vi "InitializeSettings.Do.vi"(8 "error in (no error)":errorcluster, 10 "State Variables":T9, 11 "gRPC Request":T1) -> (0 "error out":errorcluster, 2 "State Variables out":T9, 3 "gRPC Response":T6)   [LabVIEW 2025, in "xnet_can_bus_monitor_api_server_do.lvlib"]
uses:
  xnet_can_bus_monitor_api_server_do.lvlib
  Types/MainProcess.StateVariables.ctl
  Types/XNET.InitialSettings.ctl
  xnet_can_bus_monitor_api_server/RPC Messages/ni_xnet_can_bm_api_ConnectSettings.ctl
  xnet_can_bus_monitor_api_server/RPC Messages/ni_xnet_can_bm_api_CanMode.ctl
  xnet_can_bus_monitor_api_server/RPC Messages/ni_xnet_can_bm_api_Termination.ctl
  xnet_can_bus_monitor_api_server/RPC Messages/ni_xnet_can_bm_api_FdIsoMode.ctl
  xnet_can_bus_monitor_api_server/RPC Messages/ni_xnet_can_bm_api_FilterInfo.ctl
  xnet_can_bus_monitor_api_server/RPC Messages/ni_xnet_can_bm_api_DirectionFilter.ctl
  xnet_can_bus_monitor_api_server/RPC Messages/ni_xnet_can_bm_api_FrameFilter.ctl
  Types/StreamProcess.Refs.ctl
  Types/StreamProcess.VIRef.ctl
  xnet_can_bus_monitor_api_server/RPC Messages/ni_xnet_can_bm_api_InitializeSettingsReply.ctl
  xnet_can_bus_monitor_api_server/RPC Messages/ni_xnet_can_bm_api_Session.ctl
  xnet_can_bus_monitor_api_server/RPC Messages/ni_xnet_can_bm_api_ErrorInfo.ctl
  xnet_can_bus_monitor_api_server/RPC Messages/ni_xnet_can_bm_api_InitializeSettingsRequest.ctl
  <vilib>/xnet/xnet.llb/XNET Create Session (Frame Output Stream).vi
  xnet_can_bus_monitor_api_server/xnet_can_bus_monitor_api_server.lvlib
  <resource>/objmgr/xnet.rc
  <vilib>/numeric/Random Number (Range) U64.vi
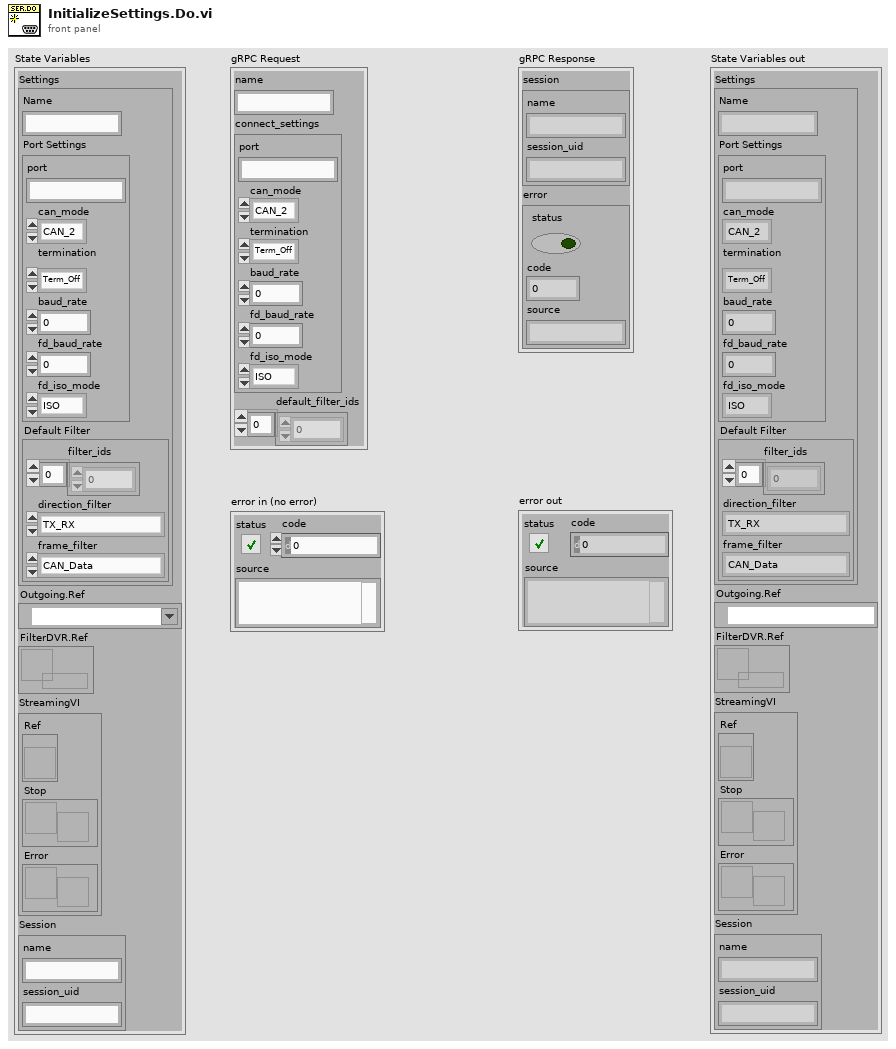
[diagram p1: front panel]
types:
  T1 = typedef "xnet_can_bus_monitor_api_server.lvlib/ni_xnet_can_bm_api_InitializeSettingsRequest.ctl" = cluster{"name":string, "connect_settings":T2, "default_filter_ids":u32[]}
  T2 = typedef "xnet_can_bus_monitor_api_server.lvlib/ni_xnet_can_bm_api_ConnectSettings.ctl" = cluster{"port":string, "can_mode":T3, "termination":T4, "baud_rate":u64, "fd_baud_rate":u64, "fd_iso_mode":T5}
  T3 = typedef "xnet_can_bus_monitor_api_server.lvlib/ni_xnet_can_bm_api_CanMode.ctl" = enum32{"CAN_2", "CAN_FD", "CAN_FD_BRS"}
  T4 = typedef "xnet_can_bus_monitor_api_server.lvlib/ni_xnet_can_bm_api_Termination.ctl" = enum32{"Term_Off", "Term_On"}
  T5 = typedef "xnet_can_bus_monitor_api_server.lvlib/ni_xnet_can_bm_api_FdIsoMode.ctl" = enum32{"ISO", "Non_ISO", "ISO_Legacy"}
  T6 = typedef "xnet_can_bus_monitor_api_server.lvlib/ni_xnet_can_bm_api_InitializeSettingsReply.ctl" = cluster{"session":T7, "error":T8}
  T7 = typedef "xnet_can_bus_monitor_api_server.lvlib/ni_xnet_can_bm_api_Session.ctl" = cluster{"name":string, "session_uid":string}
  T8 = typedef "xnet_can_bus_monitor_api_server.lvlib/ni_xnet_can_bm_api_ErrorInfo.ctl" = errorcluster
  T9 = typedef "xnet_can_bus_monitor_api_server_do.lvlib/MainProcess.StateVariables.ctl" = cluster{"Settings":T10, "Outgoing.Ref":refnum<k21>, "FilterDVR.Ref":refnum<data-value>, "StreamingVI":T14, "Session":T7}
  T10 = typedef "xnet_can_bus_monitor_api_server_do.lvlib/XNET.InitialSettings.ctl" = cluster{"Name":string, "Port Settings":T2, "Default Filter":T11}
  T11 = typedef "xnet_can_bus_monitor_api_server.lvlib/ni_xnet_can_bm_api_FilterInfo.ctl" = cluster{"filter_ids":u32[], "direction_filter":T12, "frame_filter":T13}
  T12 = typedef "xnet_can_bus_monitor_api_server.lvlib/ni_xnet_can_bm_api_DirectionFilter.ctl" = enum32{"TX_RX", "RX", "TX"}
  T13 = typedef "xnet_can_bus_monitor_api_server.lvlib/ni_xnet_can_bm_api_FrameFilter.ctl" = enum32{"CAN_Data", "CAN_Remote", "CAN_Bus_Error", "CAN_2_Data", "CAN_FD_Data", "CAN_FD_BRS_Data", "J1939_Data", "Delay", "Log_Trigger", "Start_Trigger", "All"}
  T14 = typedef "xnet_can_bus_monitor_api_server_do.lvlib/StreamProcess.Refs.ctl" = cluster{"Ref":T15, "Stop":refnum<notifier>, "Error":refnum<notifier>}
  T15 = typedef "xnet_can_bus_monitor_api_server_do.lvlib/StreamProcess.VIRef.ctl" = refnum<vi>
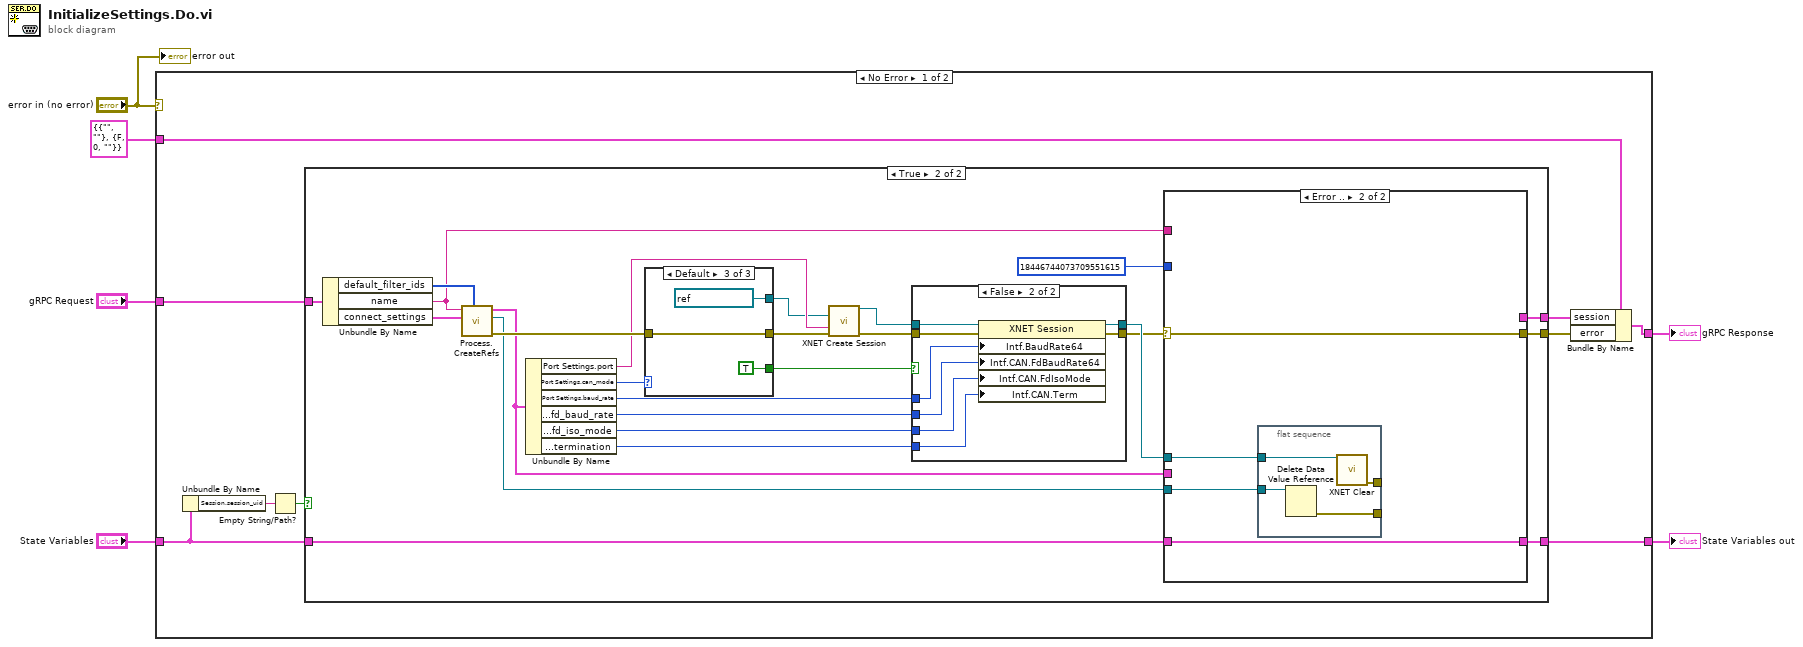
[diagram p0: block diagram]
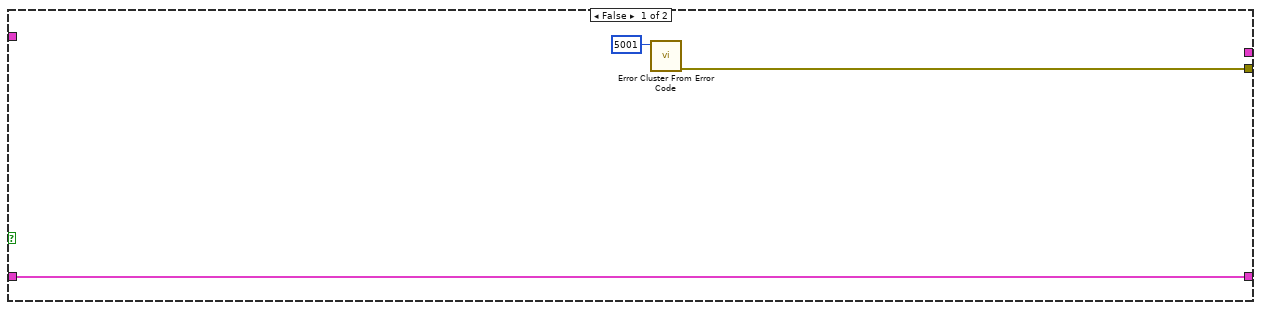
[diagram p2: hidden frame]
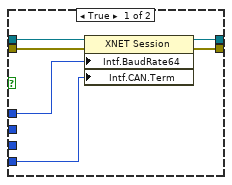
[diagram p3: hidden frame]
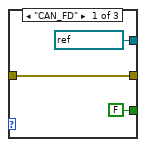
[diagram p4: hidden frame]
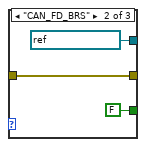
[diagram p5: hidden frame]
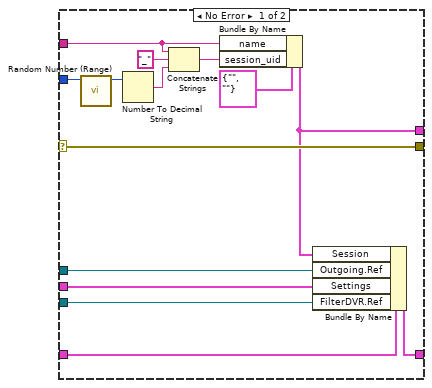
[diagram p6: hidden frame]
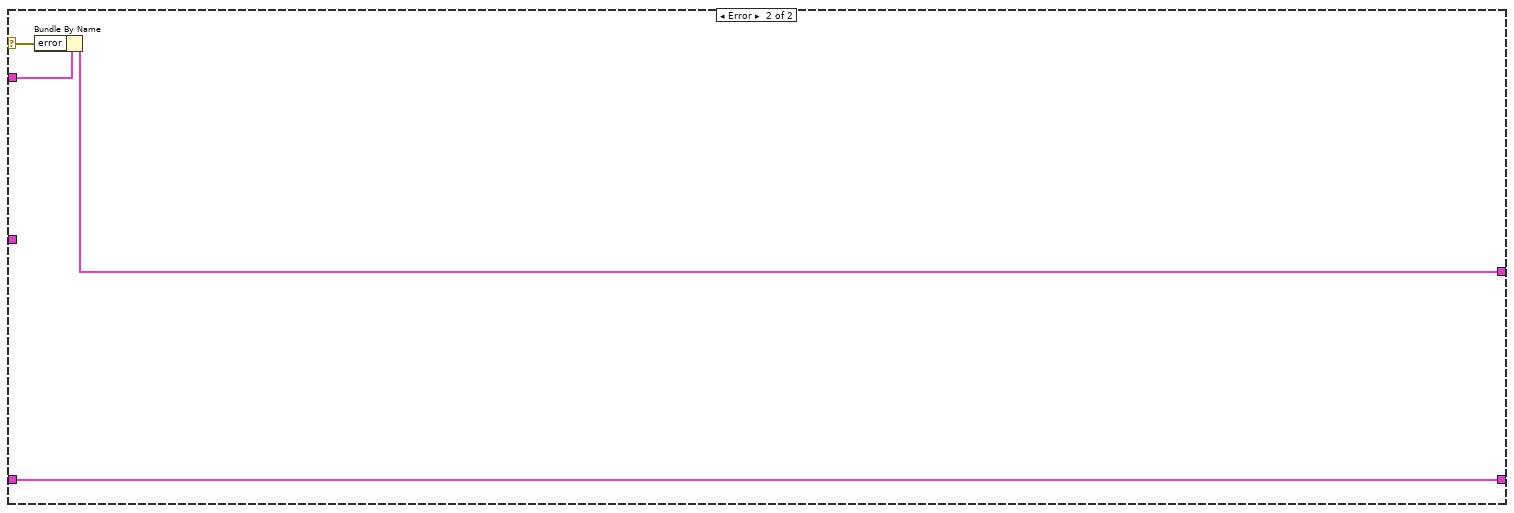
[diagram p7: hidden frame]
diagram:
  n1 = case shown="No Error" "error in (no error)" {
    selector: "error in (no error)" -> [_ w90]
    tunnel: "State Variables" -> [w14 w92]
    tunnel: [w13 w92] -> w5
    tunnel: [w10 w89] -> w4
    tunnel: "gRPC Request" -> [w9 _]
    tunnel: T6 {"session"={"name"="", "session_uid"=""}, "error"={"status"=FALSE, "code"=0, "source"=""}} ("Message Data") -> [w8 w91]
    frame No Error {
      n2 = Unbundle By Name(w14) -> ("Session.session_uid"=w15:string)
      n3 = Empty String/Path?(string/path=w15) -> (empty?=w12:bool)
      n4 = case shown="True" w12 {
        tunnel: w9 -> [_ w43]
        tunnel: [w18 w25] -> w13
        tunnel: [w17 w22] -> w11
        tunnel: w14 -> [w18 w29]
        tunnel: [_ w21] -> w7
        frame False {
          n5 = call <vilib>:"Error Cluster From Error Code.vi"("error code (0)"=5001) -> ("error out"=w17:errorcluster)  [unwired: 8 in]
        }
        frame True {
          n6 = Unbundle By Name(w43) -> ("default_filter_ids"=w24:u32[], "name"=w20:string, "connect_settings"=w42:T2)
          n7 = call "Process.CreateRefs.vi"("Default IDs"=w24, "Port Settings"=w42, "Name"=w20) -> ("error out"=w41:errorcluster, "FilterDVR.Ref"=w27:refnum<data-value>, "Initial Settings"=w28:T10)  [unwired: 6 in]
          n8 = Unbundle By Name(w28) -> ("Port Settings.port"=w40:string, "Port Settings.can_mode"=w37:T3, "Port Settings.baud_rate"=w38:u64, "Port Settings.fd_baud_rate"=w39:u64, "Port Settings.fd_iso_mode"=w36:T5, "Port Settings.termination"=w32:T4)
          n9 = case shown="Default" w37 {
            tunnel: [refnum<k21> ":can_fd:" ("cluster (:memory:)") refnum<k21> ":can_fd_brs:" ("cluster (:memory:)") refnum<k21> ":memory:" ("cluster (:memory:)")] -> w33
            tunnel: w41 -> [w58 w61 w64]
            tunnel: [w58 w61 w64] -> w34
            tunnel: [FALSE FALSE TRUE] -> w35
            frame "CAN_FD" {
            }
            frame "CAN_FD_BRS" {
            }
            frame Default {
            }
          }
          n10 = call-poly <vilib>:"XNET Create Session.vi"("cluster (:memory:)"=w33, "interface"=w40, "error in (no error)"=w34) -> ("session out"=w30:refnum<k21>, "error out"=w31:errorcluster)  [unwired: 11 out]
          n11 = case shown="False" w35 {
            tunnel: w30 -> [w49 w57]
            tunnel: [w48 w56] -> w26
            tunnel: w31 -> [w47 w55]
            tunnel: [w46 w54] -> w23
            tunnel: w32 -> [w44 w53]
            tunnel: w38 -> [w45 w52]
            tunnel: w36 -> [_ w51]
            tunnel: w39 -> [_ w50]
            frame True {
              n12 = property class="XNET Session"(reference=w49, error in=w47, "Intf.BaudRate64"=w45, "Intf.CAN.Term"=w44) -> (reference out=w48:refnum<k21>, error out=w46:errorcluster)
            }
            frame False {
              n13 = property class="XNET Session"(reference=w57, error in=w55, "Intf.BaudRate64"=w52, "Intf.CAN.FdBaudRate64"=w50, "Intf.CAN.FdIsoMode"=w51, "Intf.CAN.Term"=w53) -> (reference out=w56:refnum<k21>, error out=w54:errorcluster)
            }
          }
          n14 = case shown="Error .." w23 {
            selector: w23 -> [w75 w84]
            tunnel: w29 -> [w80 w81]
            tunnel: w28 -> [w79 _]
            tunnel: w27 -> [w78 w82]
            tunnel: w26 -> [w77 w83]
            tunnel: [w76 w81] -> w25
            tunnel: [w75 w84] -> w22
            tunnel: [w68 _] -> w21
            tunnel: w20 -> [w71 _]
            tunnel: u64 18446744073709551615 ("upper bound (100)") -> [w67 _]
            frame No Error {
              n15 = call-poly <vilib>:"Random Number (Range).vi"("upper bound (100)"=w67) -> ("number"=w72:u64)  [unwired: 10 in]
              n16 = Number To Decimal String(number=w72) -> (decimal integer string=w70:string)  [unwired: 1 in]
              n17 = Concatenate Strings(w71, "_" ("string"), w70) -> (w73:string)
              n18 = Bundle By Name(cluster=T7 {"name"="", "session_uid"=""} ("session"), "name"=w71, "session_uid"=w73) -> (w68:T7)
              n19 = Bundle By Name(cluster=w80, "Session"=w68, "Outgoing.Ref"=w77, "Settings"=w79, "FilterDVR.Ref"=w78) -> (w76:T9)
            }
            frame Error {
              n20 = flat-sequence {
                tunnel: w83 -> [w88]
                tunnel: w82 -> [w87]
                tunnel: [w86] -> _
                tunnel: [w85] -> _
                frame #0 {
                  n21 = Delete Data Value Reference(data value reference=w87) -> (error out=w85:errorcluster)  [unwired: 1 in, 1 out]
                  n22 = call <vilib>:"XNET Clear.vi"("session in"=w88) -> ("error out"=w86:errorcluster)  [unwired: 14 in]
                }
              }
            }
          }
        }
      }
      n23 = Bundle By Name(cluster=w8, "session"=w7, "error"=w11) -> (w10:T6)
    }
    frame Error {
      n24 = Bundle By Name(cluster=w91, "error"=w90) -> (w89:T6)
    }
  }
  "State Variables out" <- w5
  "gRPC Response" <- w4
  "error out" <- "error in (no error)"
